vi "state machine forum nov 11.vi"() -> ()   [LabVIEW 2012]
panel:
  in  "Numeric":dbl
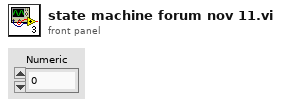
[diagram p1: front panel]
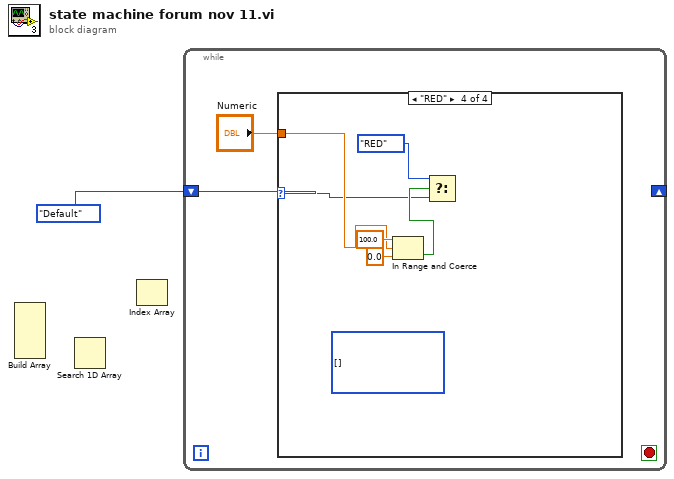
[diagram p0: block diagram]
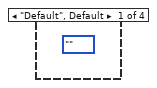
[diagram p2: hidden frame]
diagram:
  n1 = Build Array() -> ()  [unwired: 7 in, 1 out]
  n2 = Search 1D Array() -> ()  [unwired: 3 in, 1 out]
  n3 = Index Array() -> ()  [unwired: 2 in, 1 out]
  n4 = while {
    shift-right: _ -> [_]
    shift-left: enum16{"Default", "BLUE", "GREEN", "RED"}."Default" -> [w3]
    stop <- _ stop-if-true
    n5 = case shown="\"RED\"" w3 {
      selector: w3 -> [_ _ _ w4]
      tunnel: "Numeric" -> [_ _ _ w6]
      frame "Default", Default {
        (unwired) enum16{""}.""
      }
      frame "BLUE" {
      }
      frame "GREEN" {
      }
      frame "RED" {
        (unwired) enum16{"GREEN"}[] [] items=["GREEN"]
        n6 = In Range and Coerce(upper limit=100.0, x=w6, lower limit=0.0) -> (In Range?=w5:bool)  [unwired: 1 out]
        n7 = Select(t=enum16{"", "BLUE", "GREEN", "RED"}."RED", s=w5, f=w4) -> ()  [unwired: 1 out]
      }
    }
  }
